vi "labview_target.vi"() -> ()   [LabVIEW 2018]
doc: "You can use the System Exec VI to call command line utilities that return standard output to the command shell. You also can call interactive applications that you intend to launch using System Exec, but interact with using the UI of the executable."
panel:
  in  "Server IP address":string
  out "data out":string
  in  "Stop Button":bool
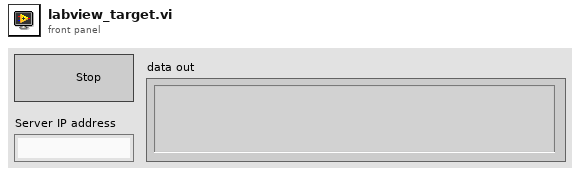
[diagram p1: front panel]
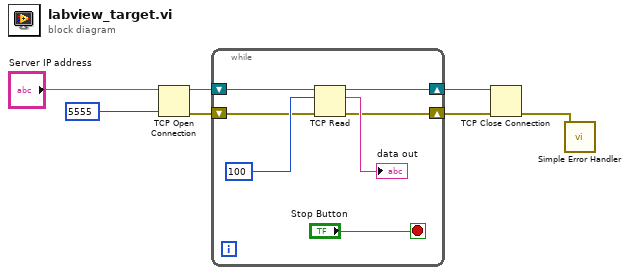
[diagram p0: block diagram]
diagram:
  n1 = TCP Open Connection(address="Server IP address", remote port or service name=5555) -> (connection ID=w2:refnum<k5>, error out=w3:errorcluster)  [unwired: 3 in]
  n2 = while {
    shift-right: [w12] -> w6
    shift-left: w3 -> [w10]
    shift-right: [w11] -> w5
    shift-left: w2 -> [w9]
    stop <- "Stop Button" stop-if-true
    n3 = TCP Read(connection ID=w9, bytes to read=100, error in (no error)=w10) -> (connection ID out=w11:refnum<k5>, data out=→"data out":string, error out=w12:errorcluster)  [unwired: 2 in]
  }
  n4 = TCP Close Connection(connection ID=w5, error in (no error)=w6) -> (error out=w4:errorcluster)  [unwired: 1 in, 1 out]
  n5 = call <vilib>:"Simple Error Handler.vi"("error in (no error)"=w4) -> ()  [unwired: 2 in, 7 out]
